vi "set digital value .vi"(9 "state":i32, 10 "pin":i32, 11 "handle":u32) -> (2 "function return":bool, 3 "handle out":u32)   [LabVIEW 2020, in "cDaq.lvlib"]
doc: "DAQAPI bool set_digital_value_(HDAQ handle, int pin, int state);"
uses:
  cDaq.lvlib
  <userlib>/cDaq/cDaq.dll
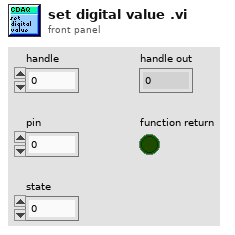
[diagram p1: front panel]
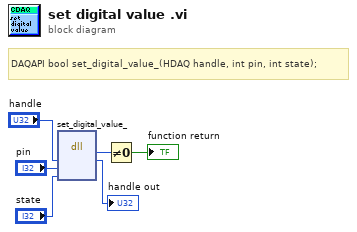
[diagram p0: block diagram]
diagram:
  # "DAQAPI bool set_digital_value_(HDAQ handle, int pin, int state);"
  n1 = dll-call lib="C:/Program Files (x86)/National Instruments/LabVIEW 2020/user.lib/cDaq/cDaq.*" fn="set_digital_value_"("handle"="handle", "pin"="pin", "state"="state") -> ("type de retour"=w5:u8, "handle"=→"handle out":u32)  [unwired: 5 in, 2 out]
  n2 = Not Equal To 0?(x=w5) -> (x != 0?=→"function return":bool)
